vi "remove from subscribers list.vi"(8 "error in (no error)":errorcluster, 10 "Subscriber Data":T1, 11 "Domino Laser module Class in":refnum<class "Domino Laser module Class.lvclass">) -> (0 "error out":errorcluster, 3 "Domino Laser module Class out":refnum<class "Domino Laser module Class.lvclass">)   [LabVIEW 2024, in "Domino LM.lvlib" / "Domino Laser module Class.lvclass"]
uses:
  CTRLS/Domino Laser module Class.lvclass
  ARCH/Message Queue/Message Cluster.ctl
  CTRLS/Domino Laser module Class.lvclass/Domino Laser module Class.ctl
  ARCH/Message Queue/Message Queue.lvlib
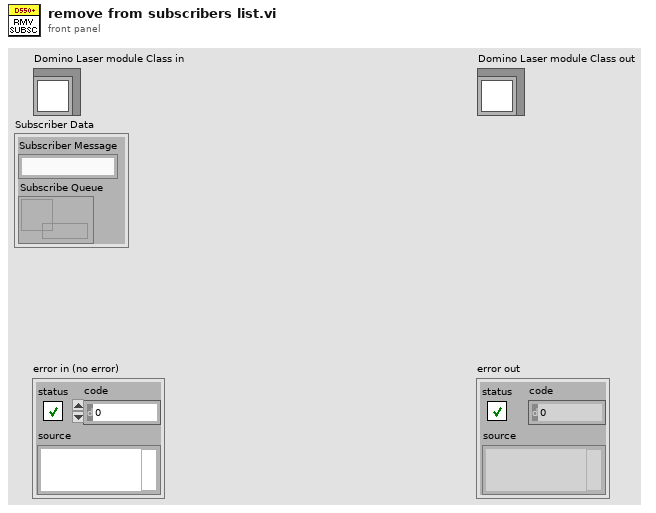
[diagram p1: front panel]
types:
  T1 = cluster{"Subscriber Message":string, "Subscribe Queue":refnum<queue>}
  T2 = cluster{"Subscriber Message":string, "Subscribe Queue":refnum<queue>}[]
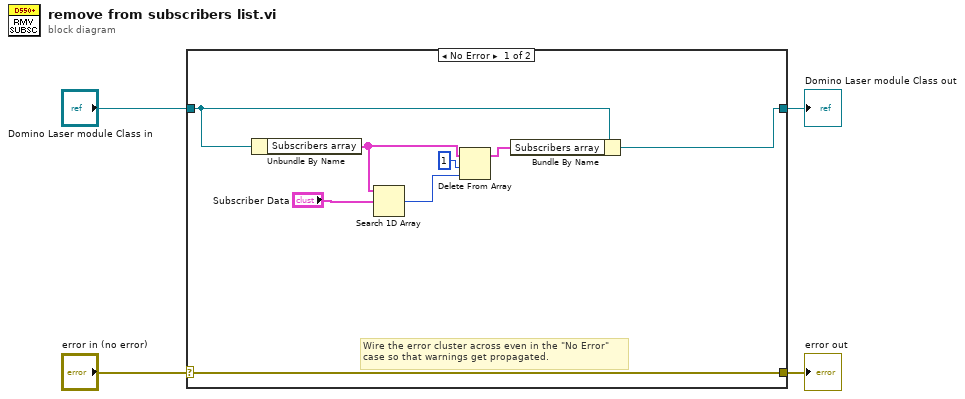
[diagram p0: block diagram]
diagram:
  n1 = case shown="No Error" "error in (no error)" {
    selector: "error in (no error)" -> [w12 w14]
    tunnel: [w12 w14] -> w3
    tunnel: [w10 w13] -> w1
    tunnel: "Domino Laser module Class in" -> [w11 w13]
    frame No Error {
      # "Wire the error cluster across even in the \"No Error\"\ncase so that warnings get propagated."
      n2 = Unbundle By Name(w11) -> ("Subscribers array"=w6:T2)
      n3 = Search 1D Array(1D array=w6, element="Subscriber Data") -> (index of element=w8:i32)  [unwired: 1 in]
      n4 = Delete From Array(array=w6, length=1, index=w8) -> (array with subset deleted=w5:T2)  [unwired: 1 out]
      n5 = Bundle By Name(cluster=w11, "Subscribers array"=w5) -> (w10:refnum<class "Domino Laser module Class.lvclass">)
    }
    frame Error {
    }
  }
  "error out" <- w3
  "Domino Laser module Class out" <- w1
